vi "getpval_v3.vi"(4 "Use Cursor":bool, 5 "Metric Choice":bool, 6 "boxsize":i32=15, 7 "amplitude":dbl[](array[numeric]), 8 "Frames number":i32=1, 9 "IntensityGraph in":refnum<vi>) -> (0 "sub-subarray":u16[][](graph), 1 "subarray":u16[][](graph), 2 "DM map":dbl[][](graph), 3 "pval":dbl)   [LabVIEW 2015]
panel:
  out "timing":u32[](array[numeric])
  out "bg":dbl
  out "I":dbl
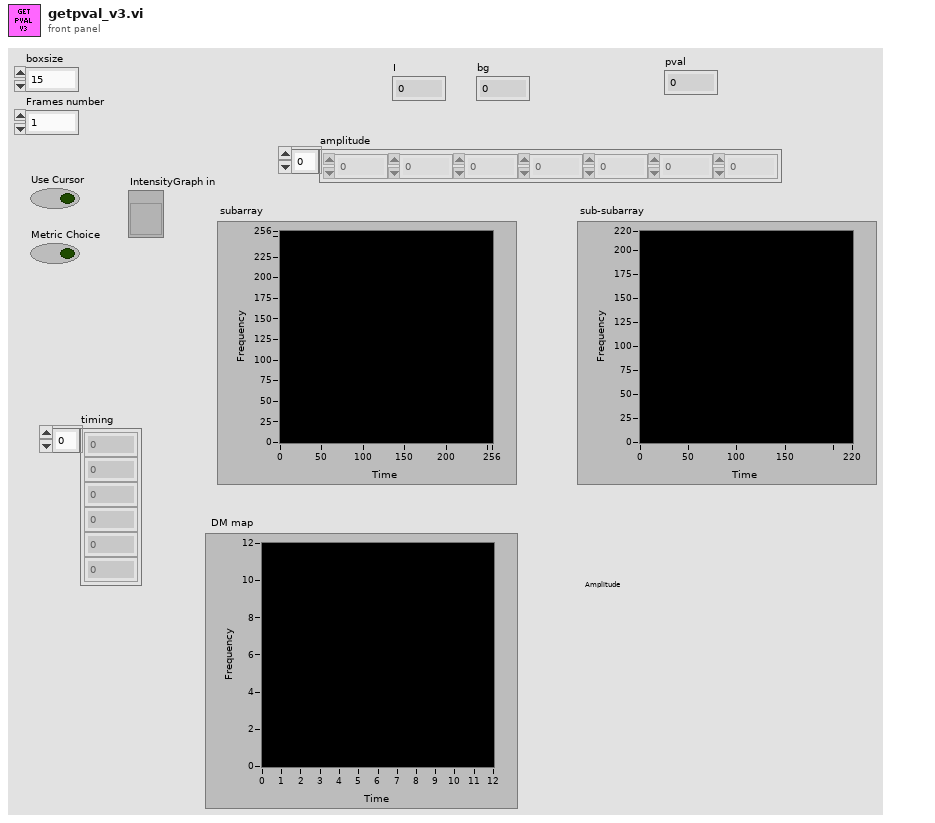
[diagram p1: front panel]
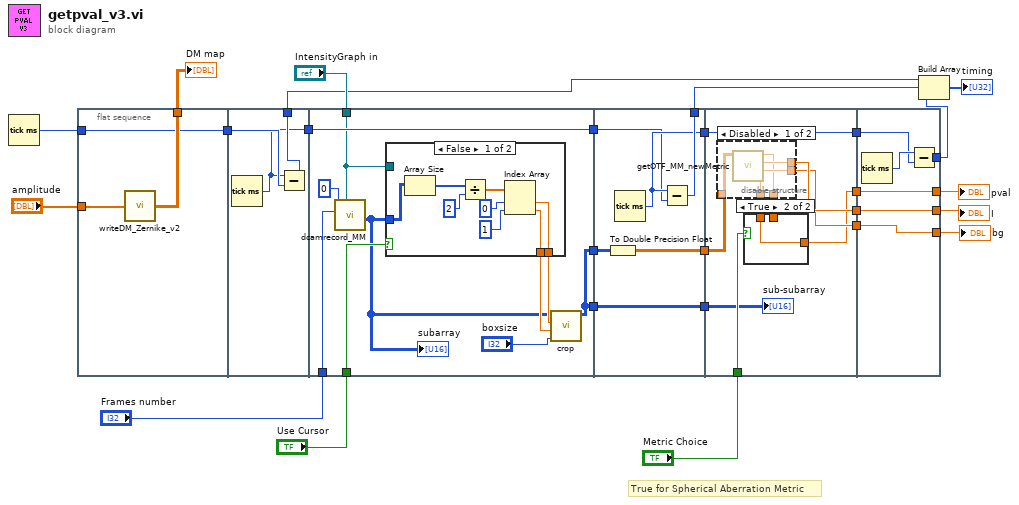
[diagram p0: block diagram]
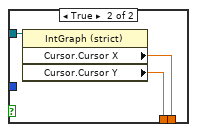
[diagram p2: hidden frame]
diagram:
  # "True for Spherical Aberration Metric"
  n1 = Tick Count (ms)() -> (millisecond timer value=w20:u32)
  n2 = flat-sequence {
    tunnel: [w29] -> w26
    tunnel: "amplitude" -> [w28]
    tunnel: w20 -> [w27]
    tunnel: [w27] -> w18
    tunnel: w18 -> [w32]
    tunnel: [w31] -> w17
    tunnel: [w30] -> w16
    tunnel: "IntensityGraph in" -> [w39]
    tunnel: [w41] -> w11
    tunnel: w16 -> [w41]
    tunnel: "Frames number" -> [w40]
    tunnel: "Use Cursor" -> [w35]
    tunnel: [w34] -> w4
    tunnel: [w34] -> w2
    tunnel: [w59] -> w9
    tunnel: [w58] -> w15
    tunnel: w11 -> [w57]
    tunnel: w4 -> [w56]
    tunnel: [w55] -> w3
    tunnel: w2 -> [w54]
    tunnel: [w54] -> w1
    tunnel: [w64] -> w14
    tunnel: [w68] -> w13
    tunnel: [w67] -> w12
    tunnel: [w66] -> w10
    tunnel: w15 -> [w66]
    tunnel: "Metric Choice" -> [w62]
    tunnel: w3 -> [w61]
    tunnel: w1 -> [w60]
    tunnel: [w79] -> w22
    tunnel: [w80] -> w23
    tunnel: [w81] -> w24
    tunnel: w14 -> [w81]
    tunnel: w13 -> [w80]
    tunnel: w12 -> [w79]
    tunnel: [w77] -> w8
    tunnel: w10 -> [w76]
    frame #0 {
      n3 = call "writeDM_Zernike_v2.vi"("amplitude"=w28) -> ("V Map Out"=w29:dbl[][])
    }
    frame #1 {
      n4 = Tick Count (ms)() -> (millisecond timer value=w30:u32)
      n5 = Subtract(x=w30, y=w32) -> (x-y=w31:u32)
    }
    frame #2 {
      n6 = call "dcamrecord_MM.vi"("IntensityGraph in"=w39, "Frames number"=w40, "Handle in"=u32 0) -> ("subarray"=w33:u16[][])  [unwired: 6 in, 2 out]
      "subarray" <- w33
      n7 = case shown="False" w35 {
        tunnel: w39 -> [_ w53]
        tunnel: [w45 w52] -> w38
        tunnel: [w44 w51] -> w37
        tunnel: w33 -> [w50 _]
        frame False {
          n8 = Array Size(array=w50) -> (size(s)=w48:i32[])
          n9 = Divide(x=w48, y=2) -> (x/y=w47:dbl[])
          n10 = Index Array(array=w47, index #1=0 ("index"), index #2=1 ("index")) -> (element #1=w45:dbl, element #2=w44:dbl)
        }
        frame True {
          n11 = property class="IntGraph (strict)"(reference=w53) -> ("Cursor.Cursor X"=w52:dbl, "Cursor.Cursor Y"=w51:dbl)  [unwired: 1 in, 2 out]
        }
      }
      n12 = call "crop.vi"("boxsize"="boxsize", "Y"=w37, "X"=w38, "Data 16"=w33) -> ("Array"=w34:u16[][])  [unwired: 7 in]
    }
    frame #3 {
      n13 = To Double Precision Float(number=w56) -> (double precision float=w55:dbl[][])
      n14 = Tick Count (ms)() -> (millisecond timer value=w58:u32)
      n15 = Subtract(x=w58, y=w57) -> (x-y=w59:u32)
    }
    frame #4 {
      n16 = disable-structure shown="Disabled" {
        disable-tunnel: [w73 _] -> w68
        disable-tunnel: [w72 _] -> w67
        disable-tunnel: [w71 _] -> w65
        disable-tunnel: [w70 _] -> w63
        disable-tunnel: w61 -> [w69 _]
        frame Disabled {
          n17 = call "getOTF_MM_newMetric.vi"("data"=w69) -> ("pval for Spherical Aberration"=w70:dbl, "bg"=w72:dbl, "I"=w73:dbl, "pval"=w71:dbl)  [unwired: 7 in]
        }
        frame Enabled {
        }
      }
      n18 = case shown="True" w62 {
        tunnel: w65 -> [w74 _]
        tunnel: [w74 w75] -> w64
        tunnel: w63 -> [_ w75]
        frame False {
        }
        frame True {
        }
      }
      "sub-subarray" <- w60
    }
    frame #5 {
      n19 = Tick Count (ms)() -> (millisecond timer value=w78:u32)
      n20 = Subtract(x=w78, y=w76) -> (x-y=w77:u32)
    }
  }
  n21 = Build Array(w17, w9, w8) -> (→"timing":u32[])
  "pval" <- w24
  "DM map" <- w26
  "I" <- w23
  "bg" <- w22
